vi "Get path (absolute).vi"(8 "error in (no error)":errorcluster, 11 "URI-Component.Path in":refnum<class "URI-Component.Path.lvclass">) -> (0 "error out":errorcluster, 2 "path-component":string, 3 "URI-Component.Path out":refnum<class "URI-Component.Path.lvclass">)   [LabVIEW 2013, in "openURI.lvlib" / "URI-Component.Path.lvclass"]
uses:
  URI-Component.Path.lvclass
  base/URI-Component.lvclass/URI-Component.ctl
  URI-Component.Path.lvclass/URI-Component.Path.ctl
  utilities/isHEXDigit.vi
  base/URI-Component.lvclass
  openURI.lvlib
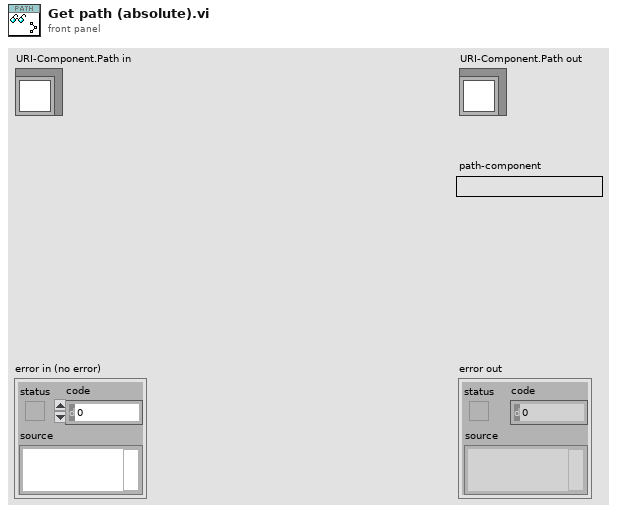
[diagram p1: front panel]
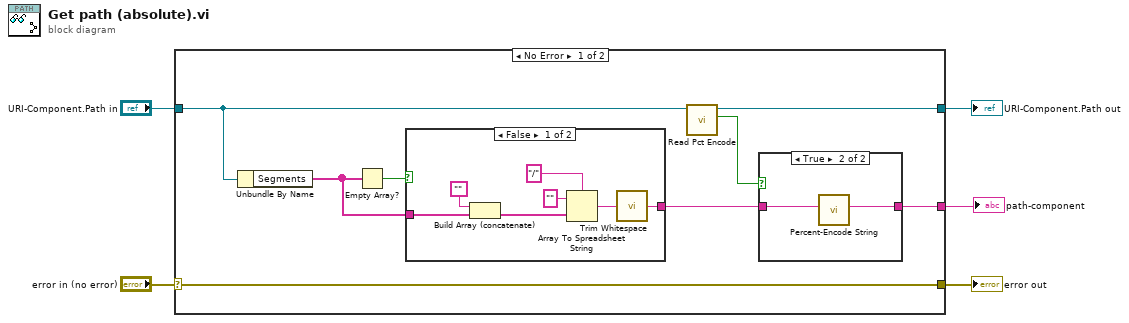
[diagram p0: block diagram]
diagram:
  n1 = case shown="No Error" "error in (no error)" {
    selector: "error in (no error)" -> [w13 w25]
    tunnel: [w13 w25] -> w4
    tunnel: [w9 w24] -> w2
    tunnel: "URI-Component.Path in" -> [w10 w24]
    tunnel: [w6 _] -> w1
    frame No Error {
      n2 = Unbundle By Name(w10) -> ("Segments"=w11:string[])
      n3 = Empty Array?(array=w11) -> (empty?=w12:bool)
      n4 = case shown="False" w12 {
        tunnel: w11 -> [w19 _]
        tunnel: [w17 _] -> w7
        frame False {
          n5 = Build Array (concatenate)("", w19) -> (w18:string[])
          n6 = Array To Spreadsheet String(delimiter (Tab)="/", array=w18, 3:"" ("format string")) -> (spreadsheet string=w21:string)
          n7 = call <vilib>:"Trim Whitespace.vi"("string"=w21) -> ("trimmed string"=w17:string)  [unwired: 1 in]
        }
        frame True {
        }
      }
      n8 = call "Read Pct Encode.vi"("URI-Component in"=w10) -> ("Pct Encode"=w8:bool, "URI-Component out"=w9:refnum<class "URI-Component.Path.lvclass">)  [unwired: 8 in, 1 out]
      n9 = case shown="True" w8 {
        tunnel: w7 -> [w14 w16]
        tunnel: [w14 w15] -> w6
        frame False {
        }
        frame True {
          n10 = call "Percent-Encode String.vi"("String"=w16) -> ("Pct-Encoded String"=w15:string)  [unwired: 10 in]
        }
      }
    }
    frame Error {
    }
  }
  "error out" <- w4
  "URI-Component.Path out" <- w2
  "path-component" <- w1
